vi "DrivePath.vi"(11 "Path":string) -> ()   [LabVIEW 2017]
uses:
  RoutineData.vi
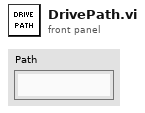
[diagram p1: front panel]
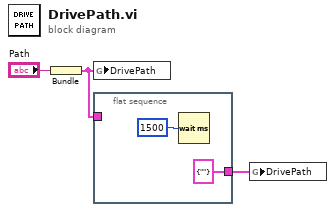
[diagram p0: block diagram]
diagram:
  n1 = Bundle("Path"="Path") -> (w3:cluster{"Path":string})  [unwired: 1 in]
  n2 = global write "RoutineData.vi" "DrivePath"(w3) -> ()
  n3 = flat-sequence {
    tunnel: w3 -> [_]
    tunnel: [cluster{"Path":string} {"Path"=""} ("DrivePath")] -> w1
    frame #0 {
      n4 = Wait (ms)(milliseconds to wait=u32 1500) -> ()  [unwired: 1 out]
    }
  }
  n5 = global write "RoutineData.vi" "DrivePath"(w1) -> ()
